vi "ReadSerial2Floats.vi"(0 "VISA resource name":refnum<visa-resource-name>, 1 "Enable":bool, 2 "baud rate (19200)":u32=9600) -> (3 "Float1":sgl, 4 "Float2":sgl, 5 "Float3":sgl, 6 "Float4":sgl)   [LabVIEW 2009]
uses:
  <vilib>/Instr/_visa.llb/VISA Configure Serial Port (Instr).vi
  <vilib>/Platform/TimedLoop/XDataNode/XDataNode.xnode
  <vilib>/Platform/TimedLoop/XDataNode/loadlvalarms.vi
  <vilib>/Platform/TimedLoop/XDataNode/timing_clust.ctl
  <vilib>/Platform/TimedLoop/XDataNode/nitl_modes.ctl
  <vilib>/Platform/TimedLoop/XDataNode/wakeup.ctl
  <vilib>/Platform/TimedLoop/XDataNode/XDNodeRunTimeDep.lvlib
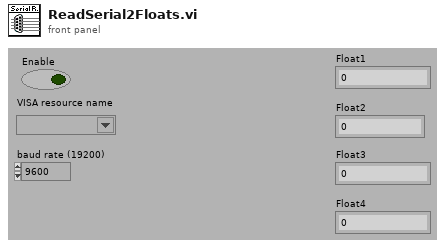
[diagram p1: front panel]
types:
  T1 = typedef "XDNodeRunTimeDep.lvlib/timing_clust.ctl" = cluster{"Expected End [f-1]":u64, "Actual End [f-1]":u64, "Finished Late? [f-1]":bool, "Expected End [i-1]":u64, "Actual End [i-1]":u64, "Finished Late? [i-1]":bool, "Expected Start [i]":u64, "Actual Start [i]":u64, "Expected Start [f]":u64, "Actual Start [f]":u64, "Source Name":string, "Structure Name":string, "Period":i64, "Deadline":i64, "Offset":i64, "Start":i64, "Priority":i32, "Timeout":i32, "Mode":T2, "Wakeup Reason":T3, "Error":errorcluster, "Source Type":string, "Secondary Source Type":string, "Global End Time":u64, "Global Start Time":u64, "Frame Duration":u64, "Iteration Duration":u64, "Assigned CPU":i32, "I/O Scan Engine Mode":u32}
  T2 = typedef "XDNodeRunTimeDep.lvlib/nitl_modes.ctl" = enum32{"No Change", "Process missed periods, maintain original phase", "Discard missed periods, maintain original phase", "Process missed periods, ignore original phase", "Discard missed periods, ignore original phase"}
  T3 = typedef "XDNodeRunTimeDep.lvlib/wakeup.ctl" = enum32{"Normal", "Aborted", "Asynchronous wakeup", "Timing source error", "Timed loop error", "Timeout"}
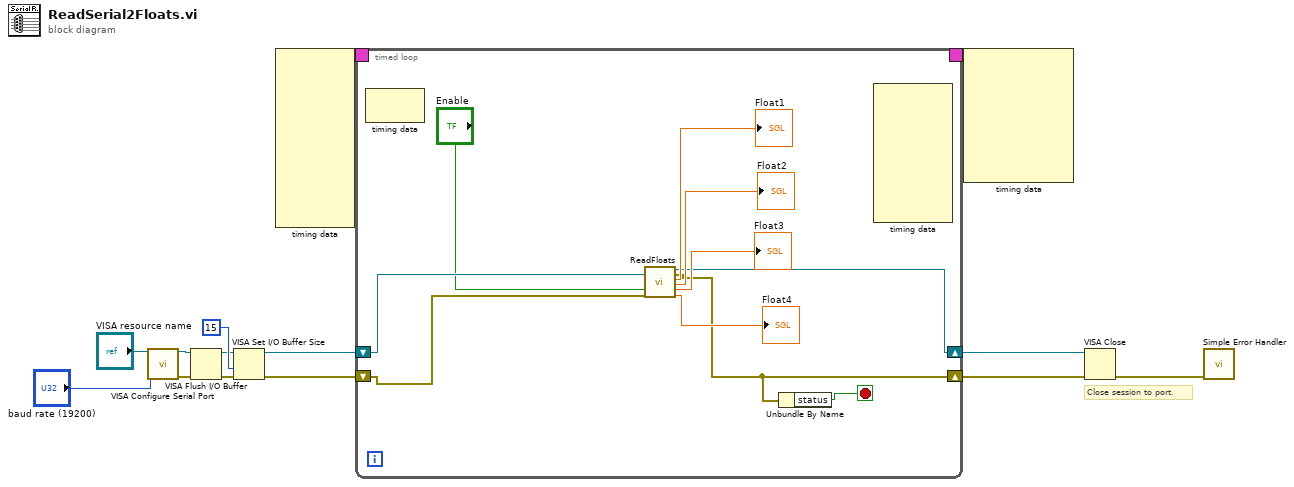
[diagram p0: block diagram]
diagram:
  # "Close session to port."
  n1 = call-poly "VISA Configure Serial Port"("VISA resource name"="VISA resource name", "baud rate (9600)"="baud rate (19200)") -> ("VISA resource name out"=w7:refnum<visa-resource-name>, "error out"=w5:errorcluster)  [unwired: 8 in, 4 out]
  n2 = VISA Flush I/O Buffer(VISA resource name=w7, error in (no error)=w5) -> (VISA resource name out=w4:refnum<visa-resource-name>, error out=w6:errorcluster)  [unwired: 1 in]
  n3 = VISA Set I/O Buffer Size(VISA resource name=w4, size (4096)=u32 15 ("baud rate (9600)"), error in (no error)=w6) -> (VISA resource name out=w3:refnum<visa-resource-name>, error out=w10:errorcluster)  [unwired: 1 in]
  n4 = node-c288() -> (w14:T1)  [unwired: 10 in]
  n5 = timed-loop {
    timing: w14 -> [_]
    timing-out: [_] -> w13
    shift-right: [w17] -> w11
    shift-left: w3 -> [w24]
    shift-right: [w16] -> w9
    shift-left: w10 -> [w19]
    stop <- w15 stop-if-true
    n6 = node-c288() -> ()  [unwired: 1 in, 1 out]
    n7 = call "ReadFloats.vi"("VISA resource name in"=w24, "Enable"="Enable", "error in"=w19) -> ("VISA resource name out"=w17:refnum<visa-resource-name>, "error out"=w16:errorcluster, "Float1"=→"Float1":sgl, "Float2"=→"Float2":sgl, "Float3"=→"Float3":sgl, "Float4"=→"Float4":sgl)  [unwired: 10 in, 1 out]
    n8 = Unbundle By Name(w16) -> ("status"=w15:bool)
    n9 = node-c288() -> ()  [unwired: 8 in, 1 out]
  }
  n10 = node-c288(w13) -> ()  [unwired: 7 out]
  n11 = VISA Close(VISA resource name=w11, error in (no error)=w9) -> (error out=w12:errorcluster)
  n12 = call <vilib>:"Simple Error Handler.vi"("error in (no error)"=w12) -> ()  [unwired: 1 in, 8 out]
